vi "PCall.vi"(4 "nresults":i32, 6 "nargs":i32, 10 "error in (no error)":errorcluster, 11 "Lua in":refnum<class "Lua.lvclass">) -> (2 "error out":errorcluster, 3 "Lua out":refnum<class "Lua.lvclass">)   [LabVIEW 2020, in "Lua for LabVIEW.lvlib" / "Lua.lvclass"]
doc: "Calls a function in protected mode.\n\nTo call a function you must use the following protocol: first, the function to be called is pushed onto the stack; then, the arguments to the function are pushed in direct order; that is, the first argument is pushed first. Finally you call lua_pcall; nargs is the number of arguments that you pushed onto the stack. All arguments and the function value are popped from the stack when the function is called. The function results are pushed onto the stack when the function returns. The number of results is adjusted to nresults, unless nresults is LUA_MULTRET. In this case, all results from the function are pushed. Lua takes care that the returned values fit into the stack space. The function results are pushed onto the stack in direct order (the first result is pushed first), so that after the call the last result is on the top of the stack."
uses:
  Lua.lvclass
  Lua.lvclass/Lua.ctl
  lib/lua.dll/lua_type.vi
  lib/lua.dll/lua_tolstring.vi
  lib/lua.dll/lua_pop.vi
  lib/lua.dll/lua_settop.vi
  lib/lua.dll/lua.dll.lvlib
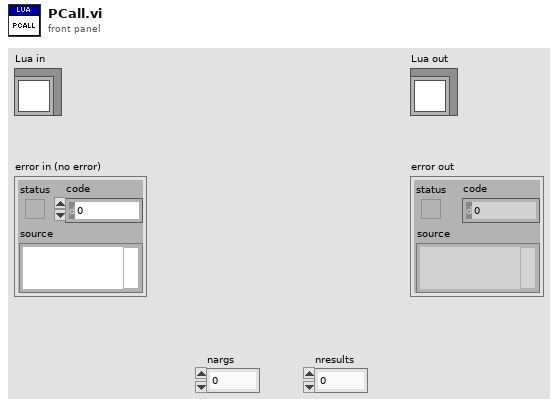
[diagram p1: front panel]
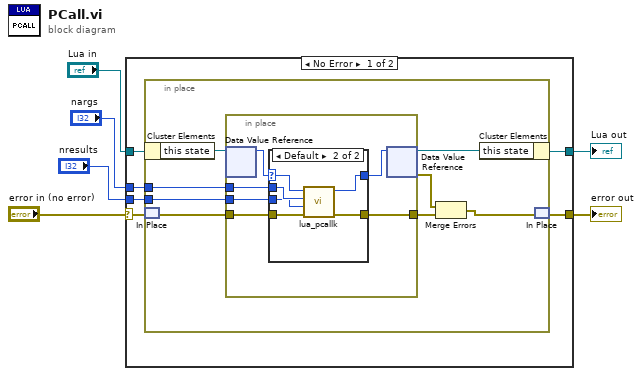
[diagram p0: block diagram]
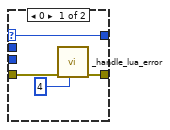
[diagram p2: hidden frame]
diagram:
  n1 = case shown="No Error" "error in (no error)" {
    selector: "error in (no error)" -> [w9 w38]
    tunnel: [w10 w38] -> w3
    tunnel: [w11 w37] -> w6
    tunnel: "Lua in" -> [w12 w37]
    tunnel: "nargs" -> [w8 _]
    tunnel: "nresults" -> [w7 _]
    frame No Error {
      n2 = in-place {
        in-place-border: w8 -> [w19]
        in-place-border: w7 -> [w18]
        n3 = in-place-cluster #1(w12) -> ("this state"=w17:refnum<data-value>)
        n4 = in-place-match #2(w9) -> (w20:errorcluster)
        n5 = in-place {
          in-place-border: w20 -> [w26]
          in-place-border: w19 -> [w25]
          in-place-border: w18 -> [w24]
          in-place-border: [w21] -> w14
          n6 = in-place-dvr #3(w17) -> (w23:u64)  [unwired: 1 out]
          n7 = case shown="Default" w23 {
            selector: w23 -> [w30 w32]
            tunnel: [w30 w36] -> w22
            tunnel: w26 -> [w27 w31]
            tunnel: [w28 w33] -> w21
            tunnel: w25 -> [_ w35]
            tunnel: w24 -> [_ w34]
            frame 0 {
              n8 = call "_handle_lua_error.vi"("lua status"=4 ("lua_load errcode"), "error in (no error)"=w27) -> ("error out"=w28:errorcluster)  [unwired: 9 in]
            }
            frame Default {
              n9 = call "lua_pcallk.vi"("error in (no error)"=w31, "nresults"=w34, "nargs"=w35, "lua_state_p"=w32) -> ("error out"=w33:errorcluster, "lua_state_p out"=w36:u64)  [unwired: 6 in]
            }
          }
          n10 = in-place-dvr #3(w22) -> (w16:refnum<data-value>, w15:errorcluster)
        }
        n11 = Merge Errors(w15, w14) -> (w13:errorcluster)
        n12 = in-place-cluster #1("this state"=w16) -> (w11:refnum<class "Lua.lvclass">)
        n13 = in-place-match #2(w13) -> (w10:errorcluster)
      }
    }
    frame Error {
    }
  }
  "error out" <- w3
  "Lua out" <- w6
